vi "GAIN command.vi"(6 "Ring":u16(ring)=1 items=["1"=1, "2"=2, "3"=3, "4"=4, "6"=0, "8"=5, "12"=6], 8 "Error In":errorcluster, 11 "SerialComm in":refnum<class "SerialComm.lvclass">) -> (0 "Error Out":errorcluster, 3 "SerialComm out":refnum<class "SerialComm.lvclass">)   [LabVIEW 2017, in "SerialComm.lvclass"]
uses:
  SerialComm.lvclass
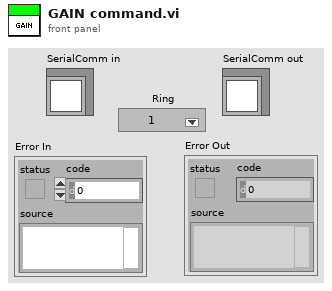
[diagram p1: front panel]
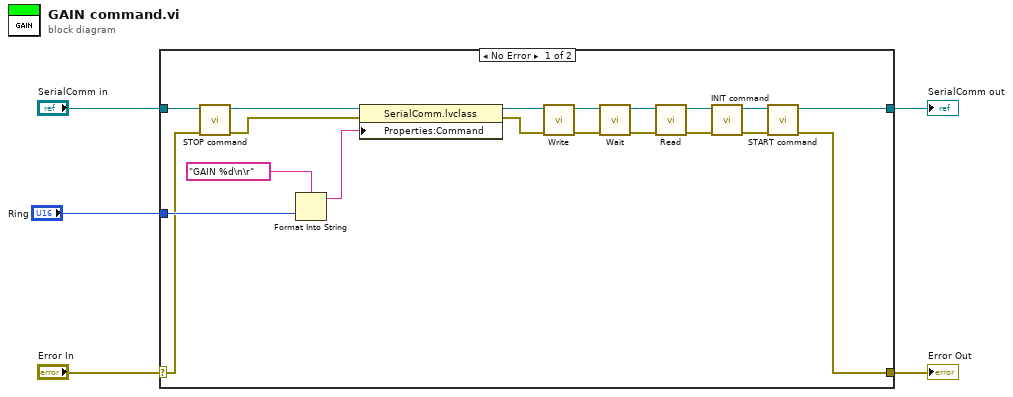
[diagram p0: block diagram]
diagram:
  n1 = case shown="No Error" "Error In" {
    selector: "Error In" -> [w13 w26]
    tunnel: [w6 w26] -> w4
    tunnel: [w7 w25] -> w2
    tunnel: "SerialComm in" -> [w18 w25]
    tunnel: "Ring" -> [w16 _]
    frame No Error {
      n2 = call "STOP command.vi"("Error In"=w13, "SerialComm in"=w18) -> ("Error Out"=w12:errorcluster, "SerialComm out"=w17:refnum<class "SerialComm.lvclass">)  [unwired: 8 in]
      n3 = Format Into String(format string="GAIN %d\n\r" ("Command"), w16) -> (resulting string=w14:string)  [unwired: 2 in, 1 out]
      n4 = property class="SerialComm.lvclass"(reference=w17, error in=w12, "Properties:Command"=w14) -> (reference out=w24:refnum<class "SerialComm.lvclass">, error out=w22:errorcluster)
      n5 = call "Write.vi"("Error In"=w22, "SerialComm in"=w24) -> ("Error Out"=w20:errorcluster, "SerialComm out"=w23:refnum<class "SerialComm.lvclass">)  [unwired: 8 in]
      n6 = call "Wait.vi"("Error In"=w20, "SerialComm in"=w23) -> ("Error Out"=w19:errorcluster, "SerialComm out"=w21:refnum<class "SerialComm.lvclass">)  [unwired: 8 in]
      n7 = call "Read.vi"("Error In"=w19, "SerialComm in"=w21) -> ("Error Out"=w11:errorcluster, "SerialComm out"=w10:refnum<class "SerialComm.lvclass">)  [unwired: 8 in]
      n8 = call "INIT command.vi"("Error In"=w11, "SerialComm in"=w10) -> ("Error Out"=w8:errorcluster, "SerialComm out"=w9:refnum<class "SerialComm.lvclass">)  [unwired: 8 in]
      n9 = call "START command.vi"("Error In"=w8, "SerialComm in"=w9) -> ("Error Out"=w6:errorcluster, "SerialComm out"=w7:refnum<class "SerialComm.lvclass">)  [unwired: 8 in]
    }
    frame Error {
    }
  }
  "Error Out" <- w4
  "SerialComm out" <- w2
